vi "ActionVIOnSave.vi"(8 "error in (no error)":errorcluster, 11 "Device Item Ref in":T1 format="%.0x") -> (0 "error out":errorcluster, 3 "Device Item Ref out":T1 format="%.0x")   [LabVIEW 2015, in "Diagnostics Addon System Explorer.lvlib"]
uses:
  Diagnostics Addon System Explorer.lvlib
  <vilib>/NI Veristand/Custom Device API/Custom Device Item Ref.ctl
  Types/FG Action.ctl
  Shared/SubVIs/GUID Lookup.vi
  <vilib>/NI Veristand/Custom Device Tools/Custom Device Utility Library/NI VeriStand - Search for Item by GUID.vi
  <vilib>/NI Veristand/Custom Device API/NI VeriStand - Set Item Property.vi
  <vilib>/NI Veristand/Custom Device API/Set Item Property (U32).vi
  <vilib>/NI Veristand/Custom Device API/NI VeriStand - Get Item Property.vi
  <vilib>/NI Veristand/Custom Device API/Get Item Property (U32).vi
  <vilib>/NI Veristand/Custom Device API/Set Item Property (U32 Array).vi
  <vilib>/NI Veristand/Custom Device API/Get Item Property (U32 Array).vi
  <vilib>/NI Veristand/Custom Device Tools/Custom Device Utility Library/Custom Device Utility Library.lvlib
  Shared/Diagnostics Addon Shared.lvlib
  <vilib>/NI Veristand/Custom Device API/Custom Device API.lvlib
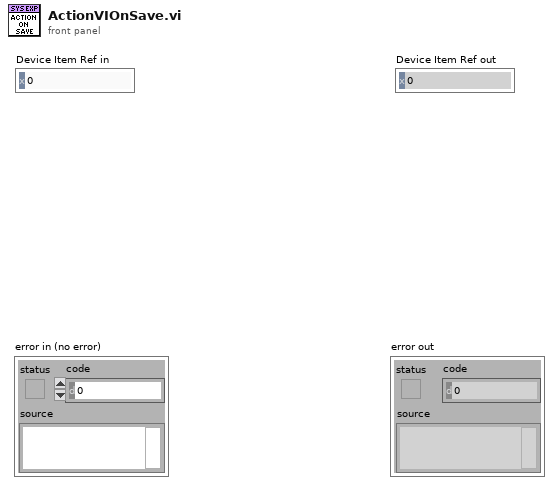
[diagram p1: front panel]
types:
  T1 = typedef "Custom Device API.lvlib/Custom Device Item Ref.ctl" = u64
  T2 = typedef "Diagnostics Addon System Explorer.lvlib/FG Action.ctl" = enum16{"Get", "Set"}
  T3 = typedef "Diagnostics Addon Shared.lvlib/DPID Parameters.ctl" = cluster{"DPID ID":u8, "Speed":T4, "PIDs":u16[]}
  T4 = typedef "Diagnostics Addon Shared.lvlib/DPID Periodic Rate.ctl" = enum16{"Slow", "Medium", "Fast"}
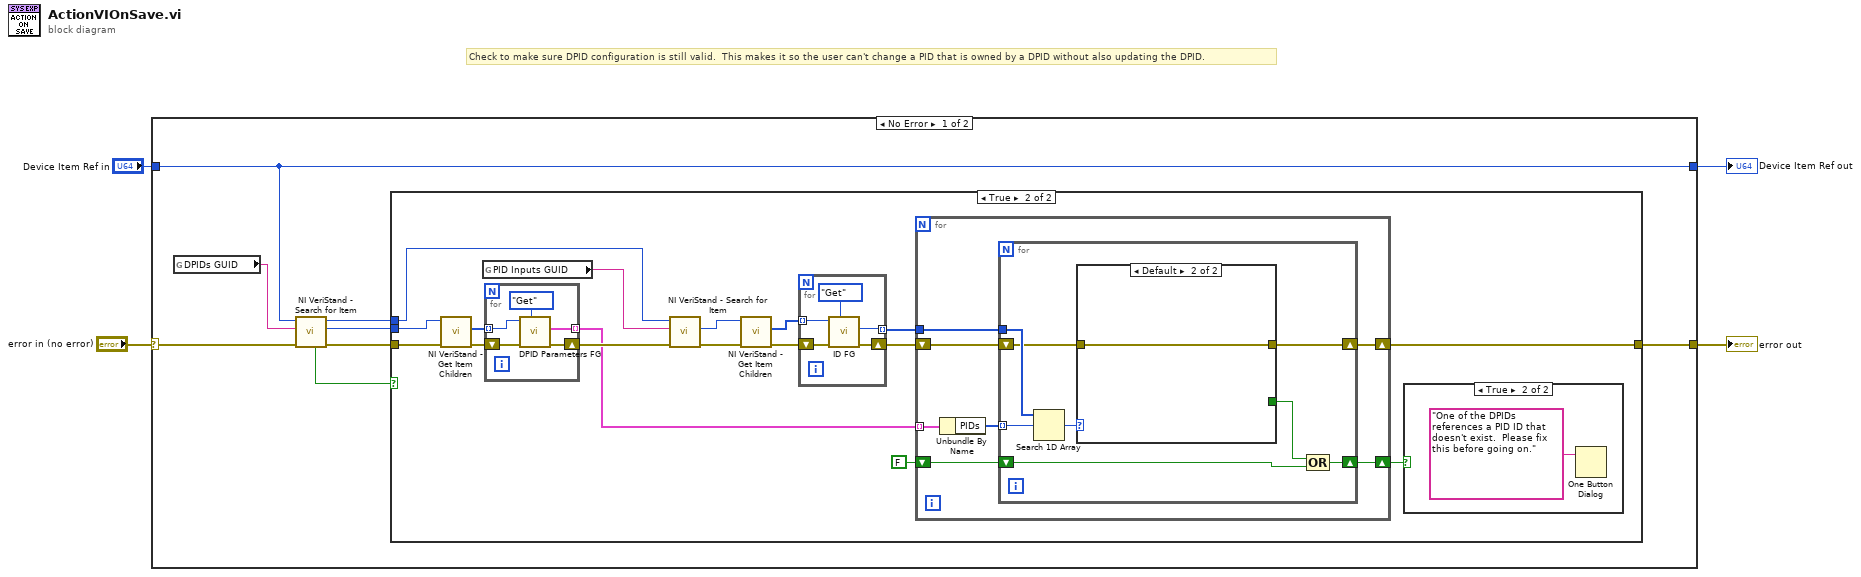
[diagram p0: block diagram]
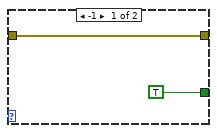
[diagram p4: hidden frame]
diagram:
  # "Check to make sure DPID configuration is still valid.  This makes it so the user can't change a PID that is owned by a DPID without also updating the DPID."
  n1 = case shown="No Error" "error in (no error)" {
    selector: "error in (no error)" -> [w12 w61]
    tunnel: [w7 w61] -> w3
    tunnel: "Device Item Ref in" -> [w5 w60]
    tunnel: [w5 w60] -> w1
    frame No Error {
      n2 = global read "GUID Lookup.vi" "DPIDs GUID"() -> (w11:string)
      n3 = call-poly <vilib>:"NI VeriStand - Search for Item.vi"("error in"=w12, "Item GUID"=w11, "Section Ref in"=w5) -> ("error out"=w8:errorcluster, "Item Ref"=w9:T1, "Section Ref out"=w6:T1, "Found"=w10:bool)  [unwired: 5 in]
      n4 = case shown="True" w10 {
        tunnel: w9 -> [_ w29]
        tunnel: w8 -> [w13 w30]
        tunnel: [w13 w16] -> w7
        tunnel: w6 -> [_ w15]
        frame False {
        }
        frame True {
          n5 = call <vilib>:"NI VeriStand - Get Item Children.vi"("error in (no error)"=w30, "Item Ref in"=w29) -> ("error out"=w28:errorcluster, "Child Refs"=w27:T1[])  [unwired: 6 in, 2 out]
          n6 = global read "GUID Lookup.vi" "PID Inputs GUID"() -> (w25:string)
          n7 = for {
            tunnel: w27 -> [w58] mode=indexing
            shift-right: [w57] -> w26
            shift-left: w28 -> [w59]
            tunnel: [w56] -> w19 mode=indexing
            n8 = call "DPID Parameters FG.vi"("Action"=FG_Action."Get", "error in (no error)"=w59, "Device Item Ref in"=w58) -> ("error out"=w57:errorcluster, "DPID"=w56:T3)  [unwired: 6 in, 1 out]
          }
          n9 = call-poly <vilib>:"NI VeriStand - Search for Item.vi"("error in"=w26, "Item GUID"=w25, "Section Ref in"=w15) -> ("error out"=w24:errorcluster, "Item Ref"=w23:T1)  [unwired: 5 in, 2 out]
          n10 = call <vilib>:"NI VeriStand - Get Item Children.vi"("error in (no error)"=w24, "Item Ref in"=w23) -> ("error out"=w22:errorcluster, "Child Refs"=w21:T1[])  [unwired: 6 in, 2 out]
          n11 = for {
            tunnel: w21 -> [w54] mode=indexing
            shift-right: [w52] -> w18
            shift-left: w22 -> [w53]
            tunnel: [w51] -> w20 mode=indexing
            n12 = call "ID FG.vi"("Action"=FG_Action."Get", "error in (no error)"=w53, "Device Item Ref in"=w54) -> ("error out"=w52:errorcluster, "ID"=w51:u32)  [unwired: 6 in, 1 out]
          }
          n13 = for {
            tunnel: w20 -> [w38]
            tunnel: w19 -> [w37] mode=indexing
            shift-right: [w32] -> w16
            shift-left: w18 -> [w35]
            shift-right: [w33] -> w14
            shift-left: FALSE -> [w34]
            n14 = Unbundle By Name(w37) -> ("PIDs"=w36:u16[])
            n15 = for {
              tunnel: w36 -> [w42] mode=indexing
              shift-right: [w43] -> w32
              shift-left: w35 -> [w44]
              tunnel: w38 -> [w46]
              shift-right: [w40] -> w33
              shift-left: w34 -> [w39]
              n16 = Search 1D Array(1D array=w46, element=w42) -> (index of element=w45:i32)  [unwired: 1 in]
              n17 = case shown="Default" w45 {
                tunnel: [w48 w49] -> w43
                tunnel: w44 -> [w48 w49]
                tunnel: [TRUE _] -> w41
                frame -1 {
                }
                frame Default {
                }
              }
              n18 = Compound Arithmetic op=OR(w41, w39) -> (w40:bool)
            }
          }
          n19 = case shown="True" w14 {
            frame False {
            }
            frame True {
              n20 = One Button Dialog(message="One of the DPIDs references a PID ID that doesn't exist.  Please fix this before going on.") -> ()  [unwired: 1 in, 1 out]
            }
          }
        }
      }
    }
    frame Error {
    }
  }
  "error out" <- w3
  "Device Item Ref out" <- w1
